vi "Wrap proxy config.vi"(6 "PROXY CONFIGURATION":T1(array[cluster]), 7 "PORT CONFIGURATION":T3(array[cluster])=[{"Name"="ENET1", "IPv4 Address"="192.168.1.3", "IPv4 Subnet Mask"="255.255.255.0", "IPv6 Address"="", "is tagged?"=FALSE, "VLAN ID"=0}], 8 "error in":errorcluster, 10 "DUT Info":T2={"DUT IP"="192.168.1.12", "DUT Username"="Administrator", "DUT Password"="NITEST", "DUT SSH PORT"=22, "DUT FWD TEST PORT"=62000, "DUT MAC ADDRESS"="02:00:08:38:2d:37"}, 11 "XNET INTERFACE":string="ENET1") -> (0 "error out":errorcluster, 3 "config":string)   [LabVIEW 2026]
uses:
  DUT Info.ctl
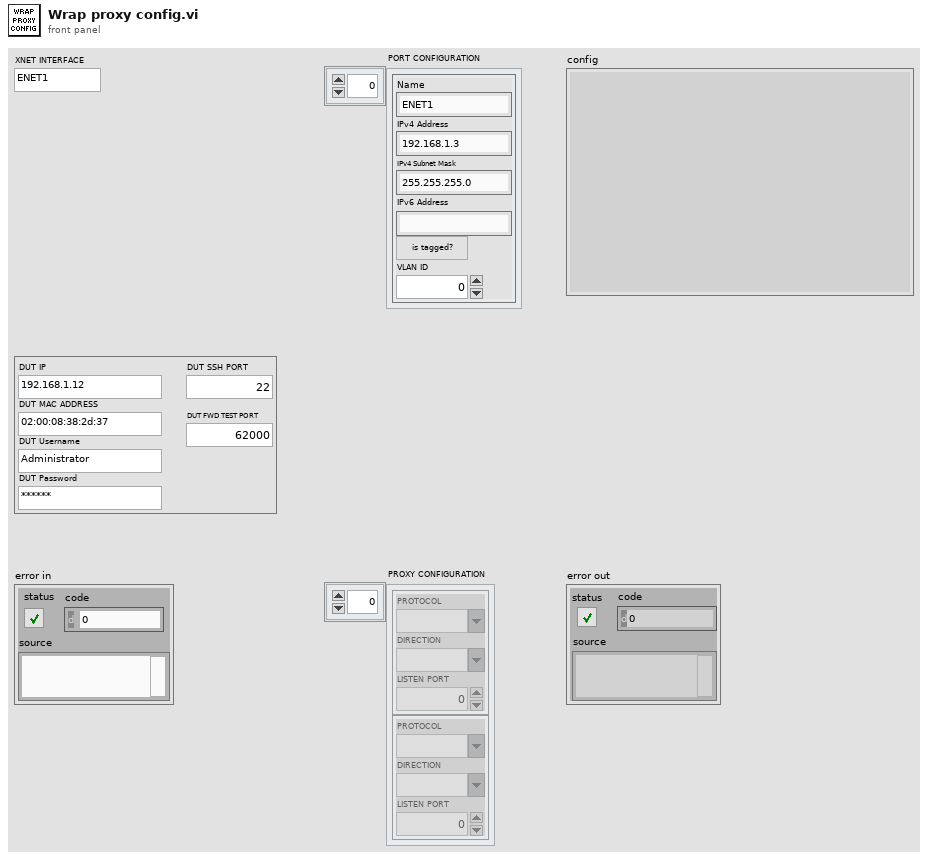
[diagram p1: front panel]
types:
  T1 = cluster{"LISTEN PORT":u16, "DIRECTION":string, "PROTOCOL":string}[]
  T2 = typedef "DUT Info.ctl" = cluster{"DUT IP":string, "DUT Username":string, "DUT Password":string, "DUT SSH PORT":u16, "DUT FWD TEST PORT":u16, "DUT MAC ADDRESS":string}
  T3 = cluster{"Name":string, "IPv4 Address":string, "IPv4 Subnet Mask":string, "IPv6 Address":string, "is tagged?":bool, "VLAN ID":u16}[]
  T4 = cluster{"Name":string, "IPv4 Address":string, "IPv4 Subnet Mask":string, "IPv6 Address":string, "is tagged?":bool, "VLAN ID":u16}
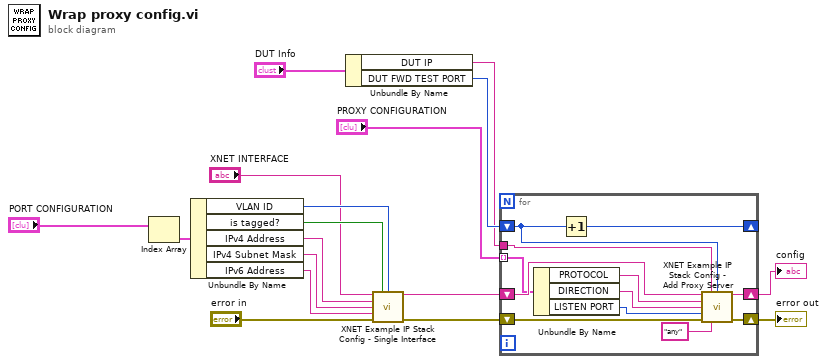
[diagram p0: block diagram]
diagram:
  n1 = Index Array(array="PORT CONFIGURATION") -> (element=w17:T4)  [unwired: 1 in]
  n2 = Unbundle By Name(w17) -> ("VLAN ID"=w12:u16, "is tagged?"=w13:bool, "IPv4 Address"=w16:string, "IPv4 Subnet Mask"=w15:string, "IPv6 Address"=w14:string)
  n3 = Unbundle By Name("DUT Info") -> ("DUT IP"=w9:string, "DUT FWD TEST PORT"=w10:u16)
  n4 = call <vilib>:"XNET Example IP Stack Config - Single Interface.vi"("XNET interface"="XNET INTERFACE", "is tagged?"=w13, "VLAN ID"=w12, "IPv4 address"=w16, "IPv4 subnet mask"=w15, "IPv6 address"=w14, "error in (no error)"="error in") -> ("config"=w11:string, "error out"=w3:errorcluster)  [unwired: 7 in]
  n5 = for {
    tunnel: w9 -> [w28]
    shift-right: [w26] -> w8
    shift-left: w11 -> [w29]
    tunnel: "PROXY CONFIGURATION" -> [w25] mode=indexing
    shift-right: [w20] -> _
    shift-left: w10 -> [w21]
    shift-right: [w19] -> w1
    shift-left: w3 -> [w18]
    n6 = Unbundle By Name(w25) -> ("PROTOCOL"=w24:string, "DIRECTION"=w23:string, "LISTEN PORT"=w22:u16)
    n7 = Increment(x=w21) -> (x+1=w20:u16)
    n8 = call <vilib>:"XNET Example IP Stack Config - Add Proxy Server.vi"("config in"=w29, "forwarding destination address"=w28, "forwarding destination port"=w21, "protocol"=w24, "direction"=w23, "listen port"=w22, "error in (no error)"=w18, "listen address"="any") -> ("config out"=w26:string, "error out"=w19:errorcluster)  [unwired: 6 in]
  }
  "config" <- w8
  "error out" <- w1
